vi "CalculateY1Y2Single.vi"(8 "error in":errorcluster, 11 "MagSpecCamera in":refnum<class "MagSpecCamera.lvclass">) -> (0 "error out":errorcluster, 3 "MagSpecCamera out":refnum<class "MagSpecCamera.lvclass">)   [LabVIEW 2020, in "MagSpecCamera.lvclass"]
uses:
  MagSpecCamera.lvclass
  CameraSettings_File.ctl
  OnOffTypeDef.ctl
  Calibration_Pixel_based.ctl
  MagSpecCamera.lvclass/MagSpecCamera.ctl
panel:
  out "Waveform Graph 4":dbl[](graph)
  out "Camera Settings 2":T1
  out "y2":dbl[](graph)
  out "y1":dbl[](graph)
  out "Waveform Graph 2":dbl[](graph)
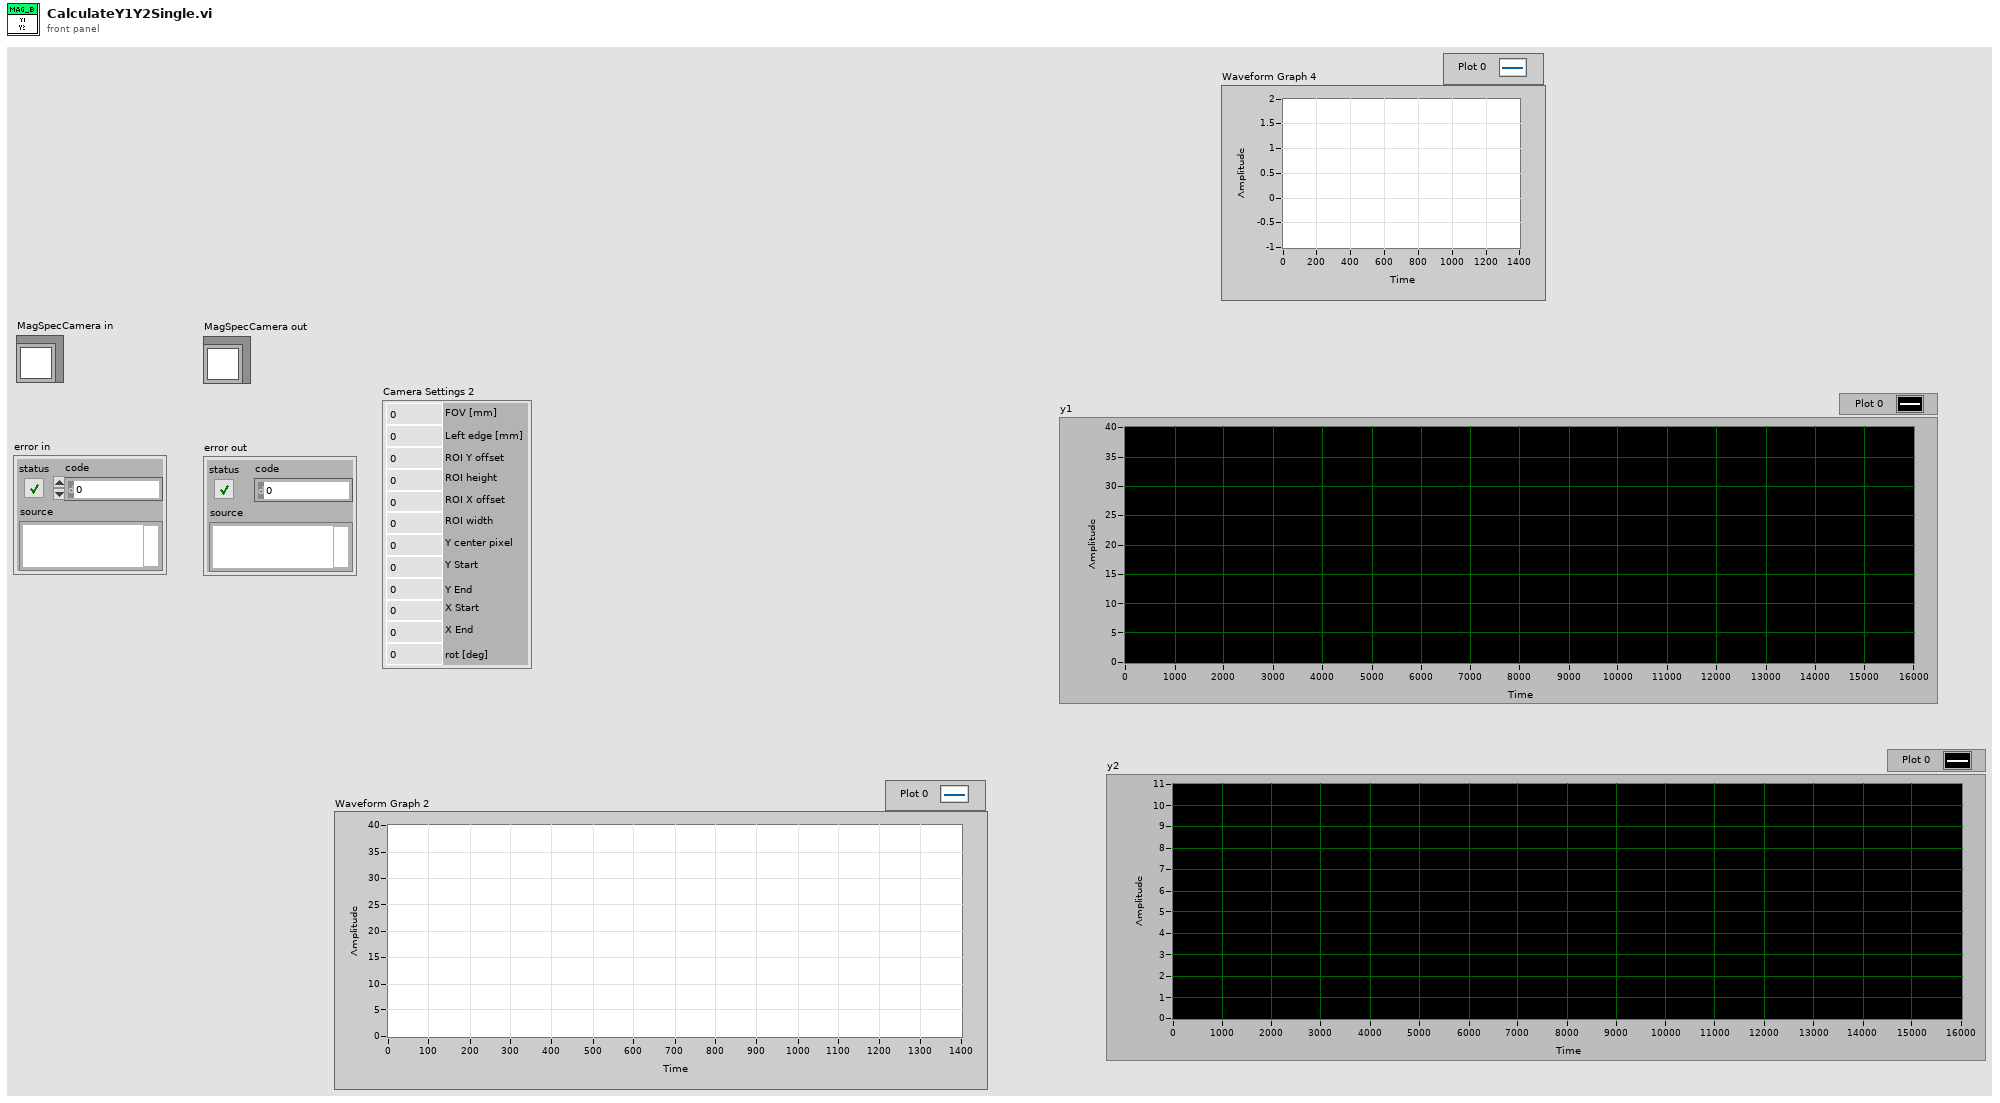
[diagram p1: front panel]
types:
  T1 = typedef "CameraSettings_File.ctl" = cluster{"FOV [mm]":dbl, "Left edge [mm]":dbl, "ROI Y offset":dbl, "ROI height":dbl, "ROI X offset":dbl, "ROI width":dbl, "Y center pixel":dbl, "Y Start":dbl, "Y End":dbl, "X Start":dbl, "X End":dbl, "rot [deg]":dbl}
  T2 = typedef "Calibration_Pixel_based.ctl" = cluster{"y1(pixel)":dbl[], "y2(pixel)":dbl[], "dp/B [MeV/C/B] (pixel)":dbl[], "energyDependence Input(pixel)":dbl[], "bending angle [deg](pixel)":dbl[], "total path(pixel)":dbl[], "pixel angle (y)(pixel)":dbl[], "energy dependence (pixel)":dbl[], "charge compensation (pixel)":dbl[], "Momentum [MeV/C](pixel)":dbl[], "angular compensation(pixel)":dbl[]}
  T3 = typedef "OnOffTypeDef.ctl" = enum16{"off", "on"}
  T4 = typedef "OneTimeCalculation.ctl" = cluster{"first Pixel pos [m]":dbl, "Pixel Size [mm]":dbl, "forward":T3}
  T5 = typedef "CalibrationCluster.ctl" = cluster{"bending angle Front":dbl[], "bending angle Side":dbl[], "screen [m] Front":dbl[], "screen [m] Side":dbl[], "momentum [MeV/c]":dbl[], "total path [m]":dbl[], "x[mm](rms)":dbl[], "x[mm](rms,b)":dbl[], "y[mm](rms)":dbl[], "y[mm](rms,b)":dbl[]}
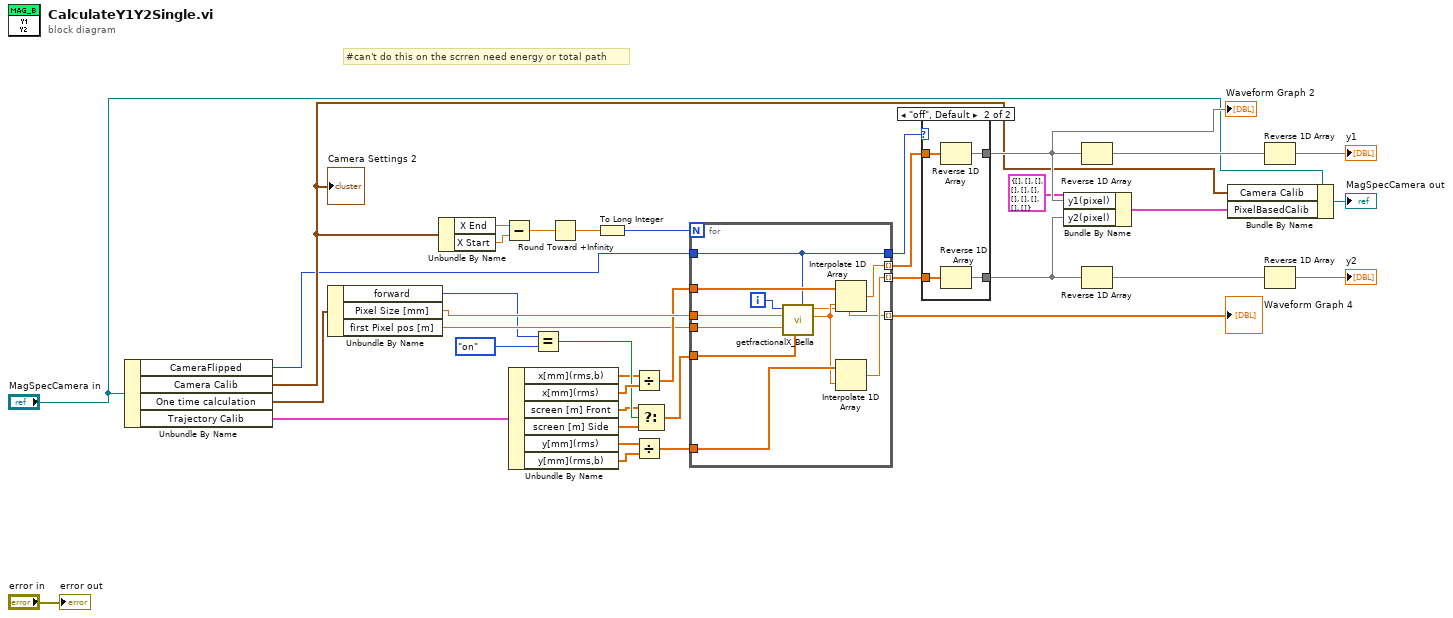
[diagram p0: block diagram]
diagram:
  # "#can't do this on the scrren need energy or total path"
  n1 = Unbundle By Name("MagSpecCamera in") -> ("CameraFlipped"=w1:T3, "Camera Calib"=w26:T1, "One time calculation"=w35:T4, "Trajectory Calib"=w36:T5)
  "Camera Settings 2" <- w26
  n2 = Unbundle By Name(w35) -> ("forward"=w2:T3, "Pixel Size [mm]"=w20:dbl, "first Pixel pos [m]"=w6:dbl)
  n3 = Unbundle By Name(w26) -> ("X End"=w16:dbl, "X Start"=w15:dbl)
  n4 = Subtract(x=w16, y=w15) -> (x-y=w5:dbl)
  n5 = Unbundle By Name(w36) -> ("x[mm](rms,b)"=w14:dbl[], "x[mm](rms)"=w21:dbl[], "screen [m] Front"=w13:dbl[], "screen [m] Side"=w12:dbl[], "y[mm](rms)"=w24:dbl[], "y[mm](rms,b)"=w23:dbl[])
  n6 = Equal?(x=w2, y=OnOffTypeDef."on") -> (x = y?=w18:bool)
  n7 = Round Toward +Infinity(x=w5) -> (ceil(x): smallest int >= x=w4:dbl)
  n8 = To Long Integer(number=w4) -> (32bit integer=w3:i32)
  n9 = Divide(x=w14, y=w21) -> (x/y=w11:dbl[])
  n10 = Divide(x=w24, y=w23) -> (x/y=w22:dbl[])
  n11 = Select(t=w13, s=w18, f=w12) -> (s? t:f=w10:dbl[])
  n12 = for {
    N: w3 -> [_]
    tunnel: w10 -> [w43]
    tunnel: w20 -> [w45]
    tunnel: w6 -> [w44]
    tunnel: w11 -> [w49]
    tunnel: w22 -> [w48]
    tunnel: [w47] -> w7 mode=indexing
    tunnel: [w46] -> w8 mode=indexing
    tunnel: w1 -> [w40]
    tunnel: [w40] -> w9
    tunnel: [w39] -> w25 mode=indexing
    i -> [w41]
    n13 = call "getfractionalX_Bella.vi"("CameraFlipped"=w40, "screen [m]"=w43, "position [m]"=w44, "pixelsize"=w45, "position index"=w41) -> ("index"=w42:dbl, "position m"=w39:dbl)  [unwired: 5 in]
    n14 = Interpolate 1D Array(1:w42, 2:w49) -> (0:w47:dbl)
    n15 = Interpolate 1D Array(1:w42, 2:w48) -> (0:w46:dbl)
  }
  "Waveform Graph 4" <- w25
  n16 = case shown="\"off\", Default" w9 {
    tunnel: [w50 w55] -> w33
    tunnel: w7 -> [w50 w54]
    tunnel: [w51 w53] -> w28
    tunnel: w8 -> [w51 w52]
    frame "on" {
    }
    frame "off", Default {
      n17 = Reverse 1D Array(array=w54) -> (reversed array=w55:dbl[])
      n18 = Reverse 1D Array(array=w52) -> (reversed array=w53:dbl[])
    }
  }
  "Waveform Graph 2" <- w33
  n19 = Bundle By Name(cluster=T2 {"y1(pixel)"=[], "y2(pixel)"=[], "dp/B [MeV/C/B] (pixel)"=[], "energyDependence Input(pixel)"=[], "bending angle [deg](pixel)"=[], "total path(pixel)"=[], "pixel angle (y)(pixel)"=[], "energy dependence (pixel)"=[], "charge compensation (pixel)"=[], "Momentum [MeV/C](pixel)"=[], "angular compensation(pixel)"=[]} ("Cluster"), "y1(pixel)"=w33, "y2(pixel)"=w28) -> (w37:T2)
  n20 = Reverse 1D Array(array=w33) -> (reversed array=w30:dbl[])
  n21 = Reverse 1D Array(array=w28) -> (reversed array=w32:dbl[])
  n22 = Bundle By Name(cluster="MagSpecCamera in", "Camera Calib"=w26, "PixelBasedCalib"=w37) -> (→"MagSpecCamera out":refnum<class "MagSpecCamera.lvclass">)
  n23 = Reverse 1D Array(array=w30) -> (reversed array=→"y1":dbl[])
  n24 = Reverse 1D Array(array=w32) -> (reversed array=→"y2":dbl[])
  "error out" <- "error in"
